vi "WR PROCSSING.vi"(7 "WR":enum16{"写", "读"}(ring), 9 "标尺.范围:最大值":dbl, 11 "进度":u8(slide) scale=0.0..100.0) -> (3 "本VI":refnum<vi>)   [LabVIEW 2014]
panel:
  out "滑动杆":u8(slide) caption="参数保存中......" scale=0.0..40.0
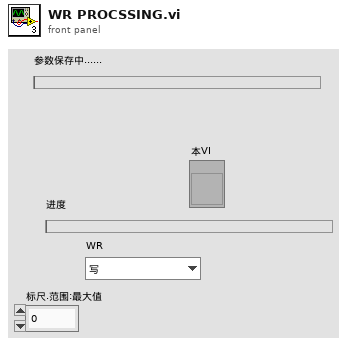
[diagram p1: front panel]
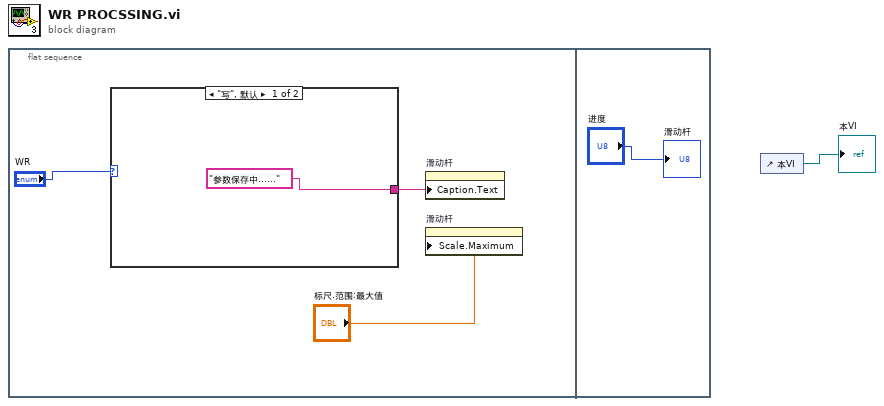
[diagram p0: block diagram]
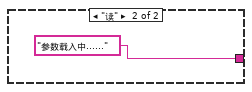
[diagram p2: hidden frame]
diagram:
  n1 = flat-sequence {
    frame #0 {
      n2 = case shown="\"写\", 默认" "WR" {
        tunnel: ["参数保存中......" ("标签.文本") "参数载入中......" ("标签.文本")] -> w3
        frame "写", Default {
        }
        frame "读" {
        }
      }
      n3 = property on="滑动杆" class="Slide (严格)"("Caption.Text"=w3) -> ()  [unwired: 2 in, 2 out]
      n4 = property on="滑动杆" class="Slide (严格)"("Scale.Maximum"="标尺.范围:最大值") -> ()  [unwired: 2 in, 2 out]
    }
    frame #1 {
      "滑动杆" <- "进度"
    }
  }
  n5 = control-ref of="本VI"() -> (→"本VI":refnum<vi>)
